vi "ProstateGlobal.vi"() -> ()   [LabVIEW 2022 SP3]
panel:
  in  "DaqMX?":bool=TRUE
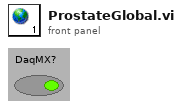
[diagram p1: front panel]
diagram:
